vi "FRCts20_WebMethods_Competition_PUT.vi"(7 "httpRequestID":u32, 11 "competition":string) -> ()   [LabVIEW 2014]
doc: "<B>PUT</B> on the specified <B>competition</B> resource\n\n<B>Required Data : </B>\n<Competition>\n <Start_Date><B>YYYY-MM-DD</B></Start_Date>\n <Duration><B>uInt</B></Duration>\n</Competition>\n\nhttp://<server address>:<port>/FRCts/competition/<B>competition</B>\n\n{requires authentication}"
uses:
  FRCts20_WebMethods.lvlib
  <vilib>/wsapi/NI_WebServices.lvlib
  Backend/source/VI Source/FRCts20_Backend_API/FRCts20_Backend_API_Competition.ctl
  Backend/source/VI Source/FRCts20_Backend_API/FRCts20_Backend_API_Command_Competition.ctl
  FRCts20_WebMethods_ReadData_Competition.vi
  Backend/source/VI Source/FRCts20_Backend_API/FRCts20_Backend_API_Application.vi
  FRCts20_WebMethods_Redirect_Request.vi
panel:
  in  "query":string
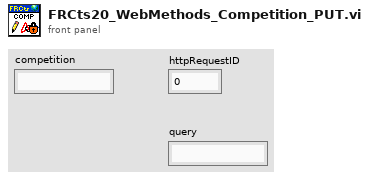
[diagram p1: front panel]
types:
  T1 = typedef "FRCts20_Backend_API.lvlib/FRCts20_Backend_API_Competition.ctl" = cluster{"Name":string, "Start Date":timestamp, "Duration":u8, "Divisions":string[], "APIReturn":string}
  T2 = typedef "FRCts20_Backend_API.lvlib/FRCts20_Backend_API_Command_Competition.ctl" = string
  T3 = typedef "FRCts20_Backend_API.lvlib/FRCts20_Backend_API_Application.ctl" = cluster{"Revision":string, "APIReturn":string}
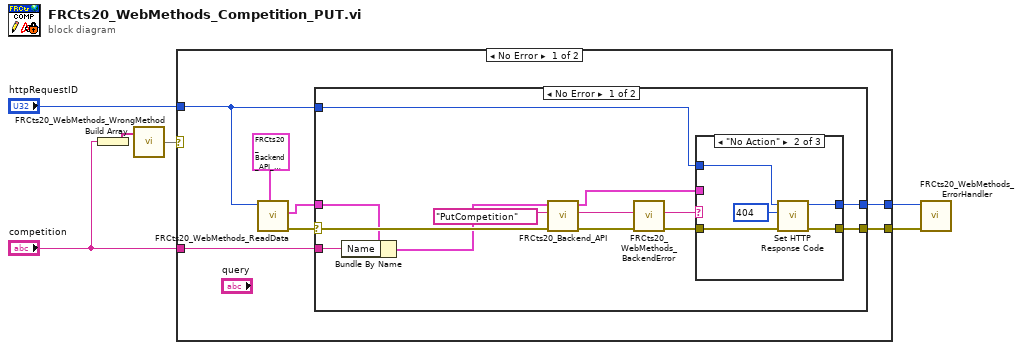
[diagram p0: block diagram]
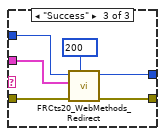
[diagram p3: hidden frame]
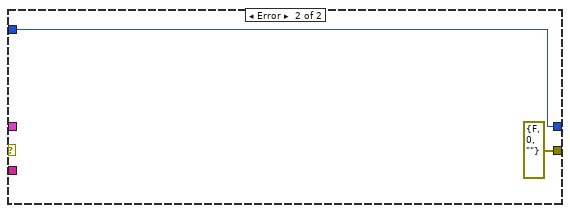
[diagram p4: hidden frame]
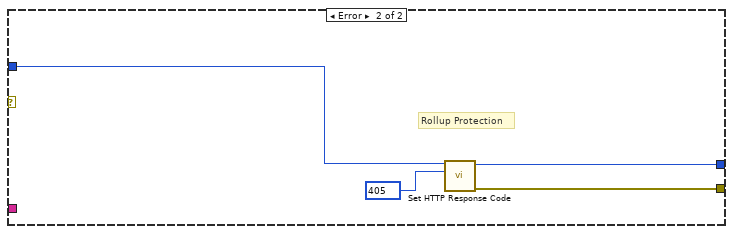
[diagram p5: hidden frame]
diagram:
  n1 = Build Array("competition") -> (w4:string[])
  n2 = call "FRCts20_WebMethods_WrongMethod.vi"(4:w4) -> (1:w5)  [unwired: 3 in, 1 out]
  n3 = case shown="No Error" w5 {
    tunnel: "httpRequestID" -> [w10 w44]
    tunnel: [w9 w43] -> w3
    tunnel: [w8 w42] -> w2
    tunnel: "competition" -> [w7 _]
    frame No Error {
      n4 = call-poly "FRCts20_WebMethods_ReadData.vi"("Competition in"=T1 {"Name"="", "Start Date"=timestamp(0 s since 1904-01-01), "Duration"=0, "Divisions"=[], "APIReturn"=""} ("Competition"), "httpRequestID"=w10) -> ("error out"=w12:errorcluster, "Competition out"=w11:T1)  [unwired: 7 in, 1 out]
      n5 = case shown="No Error" w12 {
        selector: w12 -> [w26 _]
        tunnel: w11 -> [w16 _]
        tunnel: w10 -> [w19 w41]
        tunnel: [w18 errorcluster {"status"=FALSE, "code"=0, "source"=""} ("error out")] -> w9
        tunnel: [w17 w41] -> w8
        tunnel: w7 -> [w15 _]
        frame No Error {
          n6 = Bundle By Name(cluster=w16, "Name"=w15) -> (w14:T1)
          n7 = call-poly "FRCts20_Backend_API.vi"("error in (no error)"=w26, "Command"=T2 "PutCompetition", 11:w14) -> ("error out"=w24:errorcluster, "Status"=w23:string, "Application"=w20:T3)  [unwired: 6 in]
          n8 = call "FRCts20_WebMethods_BackendError.vi"("error in (no error)"=w24, "Status"=w23) -> ("error out"=w21:errorcluster, "Status out"=w22:string)  [unwired: 8 in]
          n9 = case shown="\"No Action\"" w22 {
            tunnel: w21 -> [w27 w30 w39]
            tunnel: w20 -> [_ _ w38]
            tunnel: w19 -> [w28 w31 w37]
            tunnel: [w27 w33 w35] -> w18
            tunnel: [w28 w32 w34] -> w17
            frame "Backend Error", Default {
            }
            frame "No Action" {
              w29 = 404 items=["100"=100, "101"=101, "200"=200, "201"=201, "202"=202, "203"=203, "204"=204, "205"=205, "206"=206, "300"=300, "301"=301, "302"=302, "303"=303, "304"=304, "305"=305, "306"=306, "307"=307, "400"=400, "401"=401, "402"=402, "403"=403, "404"=404, "405"=405, "406"=406, "407"=407, "408"=408, "409"=409, "410"=410, "411"=411, "412"=412, "413"=413, "414"=414, "415"=415, "416"=416, "417"=417, "500"=500, "501"=501, "502"=502, "503"=503, "504"=504, "505"=505] ("response code (200)")
              n10 = call <vilib>:"Set HTTP Response Code.vi"("error in (no error)"=w30, "response code (200)"=w29, "httpRequestID"=w31) -> ("error out"=w33:errorcluster, "httpRequestID out"=w32:u32)  [unwired: 7 in]
            }
            frame "Success" {
              w36 = 200 items=["100"=100, "101"=101, "200"=200, "201"=201, "202"=202, "203"=203, "204"=204, "205"=205, "206"=206, "300"=300, "301"=301, "302"=302, "303"=303, "304"=304, "305"=305, "306"=306, "307"=307, "400"=400, "401"=401, "402"=402, "403"=403, "404"=404, "405"=405, "406"=406, "407"=407, "408"=408, "409"=409, "410"=410, "411"=411, "412"=412, "413"=413, "414"=414, "415"=415, "416"=416, "417"=417, "500"=500, "501"=501, "502"=502, "503"=503, "504"=504, "505"=505] ("response code (200)")
              n11 = call-poly "FRCts20_WebMethods_Redirect.vi"("response code (200)"=w36, "error in (no error)"=w39, "Request"=w38, "httpRequestID"=w37) -> ("error out"=w35:errorcluster, "httpRequestID out"=w34:u32)  [unwired: 6 in]
            }
          }
        }
        frame Error {
        }
      }
    }
    frame Error {
      w45 = 405 items=["100"=100, "101"=101, "200"=200, "201"=201, "202"=202, "203"=203, "204"=204, "205"=205, "206"=206, "300"=300, "301"=301, "302"=302, "303"=303, "304"=304, "305"=305, "306"=306, "307"=307, "400"=400, "401"=401, "402"=402, "403"=403, "404"=404, "405"=405, "406"=406, "407"=407, "408"=408, "409"=409, "410"=410, "411"=411, "412"=412, "413"=413, "414"=414, "415"=415, "416"=416, "417"=417, "500"=500, "501"=501, "502"=502, "503"=503, "504"=504, "505"=505] ("response code (200)")
      # "Rollup Protection"
      n12 = call <vilib>:"Set HTTP Response Code.vi"("response code (200)"=w45, "httpRequestID"=w44) -> ("error out"=w43:errorcluster, "httpRequestID out"=w42:u32)  [unwired: 8 in]
    }
  }
  n13 = call "FRCts20_WebMethods_ErrorHandler.vi"("error in"=w3, "LabVIEW Web Service Request"=w2) -> ()  [unwired: 8 in, 2 out]
